vi "getsubnetrange.vi"(0 "IP Address":string="255.255.255.255", 1 "Subnet Mask":string="255.255.255.255") -> (2 "Highest Usable Address":u32, 3 "Lowest Usable Address":u32, 4 "bit Mask":string)   [LabVIEW 2013]
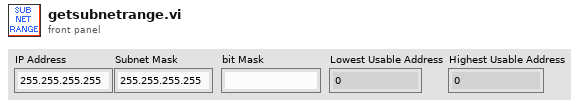
[diagram p1: front panel]
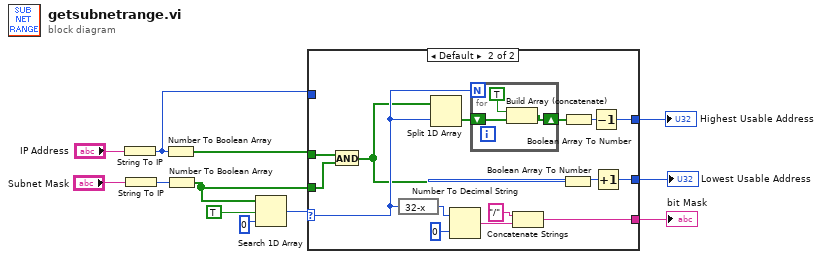
[diagram p0: block diagram]
diagram:
  n1 = String To IP(1:"IP Address") -> (0:w5:u32)
  n2 = String To IP(1:"Subnet Mask") -> (0:w7:u32)
  n3 = Number To Boolean Array(number=w5) -> (Boolean array=w2:bool[])
  n4 = Number To Boolean Array(number=w7) -> (Boolean array=w1:bool[])
  n5 = Search 1D Array(1D array=w1, element=TRUE, start index (0)=0) -> (index of element=w9:i32)
  n6 = case shown="Default" w9 {
    selector: w9 -> [_ w22]
    tunnel: w2 -> [_ w17]
    tunnel: w1 -> [_ w16]
    tunnel: ["/32" w20] -> w6
    tunnel: w5 -> [w13 _]
    tunnel: [w13 w19] -> w4
    tunnel: [w13 w18] -> w3
    frame 0 {
    }
    frame Default {
      n7 = And(x=w17, y=w16) -> (x .and. y?=w15:bool[])
      n8 = expression code="32-x"(w22) -> (w26:i32)
      n9 = Split 1D Array(array=w15, index=w22) -> (second subarray=w23:bool[])  [unwired: 1 out]
      n10 = Number To Decimal String(number=w26, width (-)=i16 0) -> (decimal integer string=w29:string)
      n11 = for {
        N: w22 -> [_]
        shift-right: [w32] -> w24
        shift-left: w23 -> [w30]
        n12 = Build Array (concatenate)(TRUE, w30) -> (w32:bool[])
      }
      n13 = Concatenate Strings("/" ("Substring"), w29) -> (w20:string)
      n14 = Boolean Array To Number(Boolean array=w15) -> (number=w25:u32)
      n15 = Boolean Array To Number(Boolean array=w24) -> (number=w21:u32)
      n16 = Decrement(x=w21) -> (x-1=w19:u32)
      n17 = Increment(x=w25) -> (x+1=w18:u32)
    }
  }
  "Highest Usable Address" <- w4
  "Lowest Usable Address" <- w3
  "bit Mask" <- w6
